vi "BC Verify Minor Frame Command.vi"(5 "Instruction ID":i32, 6 "Pointers":T1={"Major Command Pointer"=2206, "Major Data Pointer"=2206, "Minor Command Pointer"=2206, "Minor Data Pointer"=2206}, 7 "Target IC (1-8)":u8, 8 "error in (no error)":errorcluster, 11 "Bus Controller in":refnum<class "Bus Controller.lvclass">) -> (0 "error out":errorcluster, 3 "Bus Controller out":refnum<class "Bus Controller.lvclass">, 4 "Pointers out":T1={"Major Command Pointer"=2206, "Major Data Pointer"=2206, "Minor Command Pointer"=2206, "Minor Data Pointer"=2206})   [LabVIEW 2020, in "Unit Tests.lvlib" / "Bus Controller.lvclass"]
uses:
  Bus Controller.lvclass
  Data Pointers.ctl
  Frames & Messages/TypeDefs/BC Op Codes - Verbose.ctl
  Frames & Messages/TypeDefs/BC Condition Codes.ctl
  Bus Controller.lvclass/Bus Controller.ctl
  <vilib>/addons/_JKI Toolkits/Caraya/classes/Assert/Assert True.vi
  Dependencies/FPGA Interface/FPGA Interface.lvclass
  <vilib>/addons/_JKI Toolkits/Caraya/classes/Test/Test.lvclass
  BCI-1553 API.lvlib
  <vilib>/addons/_JKI Toolkits/Caraya/classes/Assert/Assert.lvclass
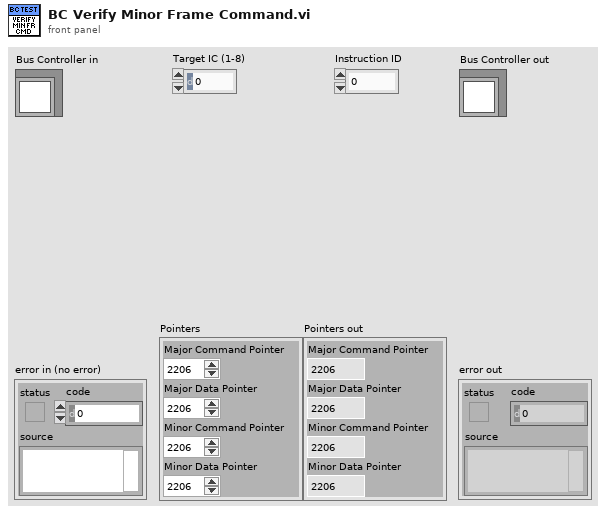
[diagram p1: front panel]
types:
  T1 = typedef "Data Pointers.ctl" = cluster{"Major Command Pointer":u16, "Major Data Pointer":u16, "Minor Command Pointer":u16, "Minor Data Pointer":u16}
  T2 = typedef "BCI-1553 API.lvlib/BC Condition Codes.ctl" = enum16{"GP0 == 1 || LT", "GP1 == 1 || NE", "GP2 == 1", "GP3 == 1", "GP4 == 1", "GP5 == 1", "GP6 == 1", "GP7 == 1", "NORESP", "FMTERR", "GOODBLOCK", "MSKSTATSET", "BADMSG", "1RETRY", "2RETRY", "ALWAYS"}
  T3 = typedef "BCI-1553 API.lvlib/BC Op Codes - Verbose.ctl" = enum16{"EXECUTE MSG", "EXECUTE MSG GO", "JUMP", "CALL SUBROUTINE", "RETURN", "INTERRUPT REQUEST", "HALT", "DELAY", "WAIT FRAME TIMER = 0", "COMPARE FRAME TIMER", "COMPARE MSG TIMER", "LOAD TIME TAG CTR", "LOAD TIME TAG CTR HI", "LOAD FRAME TIMER", "START FRAME TIMER", "PUSH TIME TAG COUNT", "PUSH TIME TAG COUNT HI", "PUSH TIME TAG COUNT BOTH", "PUSH BLOCK STATUS WORD", "PUSH CURRENT VALUE", "PUSH INDIRECT", "WAIT EXT TRIGGER", "EXECUTE AND FLIP", "EXECUTE, FLIP, GO", "WRITE VALUE TO WMI", "WRITE VALUE TO MEM", "DECREMENT RAM, SKIP", "FLAG"}
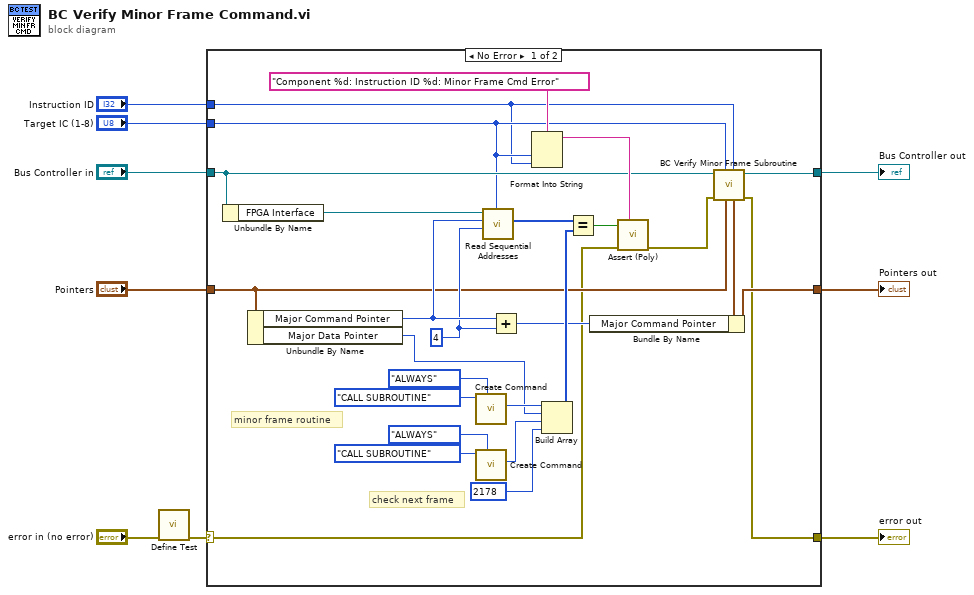
[diagram p0: block diagram]
diagram:
  n1 = call <vilib>:"Define Test.vi"("error in (no error)"="error in (no error)") -> ("error out"=w5:errorcluster)  [unwired: 9 in, 1 out]
  n2 = case shown="No Error" w5 {
    selector: w5 -> [w11 w38]
    tunnel: [w10 w38] -> w9
    tunnel: [w14 w37] -> w7
    tunnel: "Bus Controller in" -> [w20 w37]
    tunnel: "Pointers" -> [w17 _]
    tunnel: "Target IC (1-8)" -> [w19 _]
    tunnel: "Instruction ID" -> [w18 _]
    tunnel: [w15 _] -> w1
    frame No Error {
      w26 = u16 4 ("Addresses to Read")
      # "minor frame routine"
      # "check next frame"
      n3 = Unbundle By Name(w20) -> ("FPGA Interface"=w28:refnum<class "FPGA Interface.lvclass">)
      n4 = Unbundle By Name(w17) -> ("Major Command Pointer"=w27:u16, "Major Data Pointer"=w29:u16)
      n5 = call "Create Command.vi"("Condition"=BC_Condition_Codes."ALWAYS", "Op Code"=BC_Op_Codes_-_Verbose."CALL SUBROUTINE") -> ("Instruction"=w32:u16)  [unwired: 8 in, 1 out]
      n6 = call "Create Command.vi"("Condition"=BC_Condition_Codes."ALWAYS", "Op Code"=BC_Op_Codes_-_Verbose."CALL SUBROUTINE") -> ("Instruction"=w31:u16)  [unwired: 8 in, 1 out]
      n7 = call-dynamic "Read Sequential Addresses.vi"("Target IC (1-8)"=w19, "Addresses to Read"=w26, "Starting Address"=w27, "FPGA Interface in"=w28) -> ("Data"=w25:u16[])  [unwired: 6 in, 1 out]
      n8 = Add(x=w27, y=w26) -> (x+y=w16:u16)
      n9 = Format Into String(format string="Component %d: Instruction ID %d: Minor Frame Cmd Error" ("message (\"\")"), w19, w18) -> (resulting string=w21:string)  [unwired: 2 in, 1 out]
      n10 = Build Array(w32, w29, w31, u16 2178) -> (w24:u16[])
      n11 = Equal?(x=w25, y=w24) -> (x = y?=w22:bool)
      n12 = call-poly <vilib>:"Assert (Poly).vi"("Label"=w21, "error in (no error)"=w11, "True?"=w22) -> ("error out"=w12:errorcluster)  [unwired: 7 in, 1 out]
      n13 = call "BC Verify Minor Frame Subroutine.vi"("Instruction ID"=w18, "Pointers"=w17, "Target IC (1-8)"=w19, "error in (no error)"=w12, "Bus Controller in"=w20) -> ("error out"=w10:errorcluster, "Bus Controller out"=w14:refnum<class "Bus Controller.lvclass">, "Pointers out"=w13:T1)  [unwired: 4 in]
      n14 = Bundle By Name(cluster=w13, "Major Command Pointer"=w16) -> (w15:T1)
    }
    frame Error {
    }
  }
  "error out" <- w9
  "Bus Controller out" <- w7
  "Pointers out" <- w1
